vi "cam_tests.vi"() -> ()   [LabVIEW 2013]
uses:
  <vilib>/vision/driver/NI_Vision_Acquisition_Software.lvlib
  <vilib>/vision/Image Controls.llb/IMAQ Image.ctl
panel:
  out "All Images Out":T1[](array[plugin-control])
  in  "Number of Images":i32=10
  out "Image Out":T1(plugin-control)
  in  "Stop (F)":bool
  out "Image Out 2":T1(plugin-control)
  out "error out":errorcluster
  out "Image 3":T1(plugin-control)
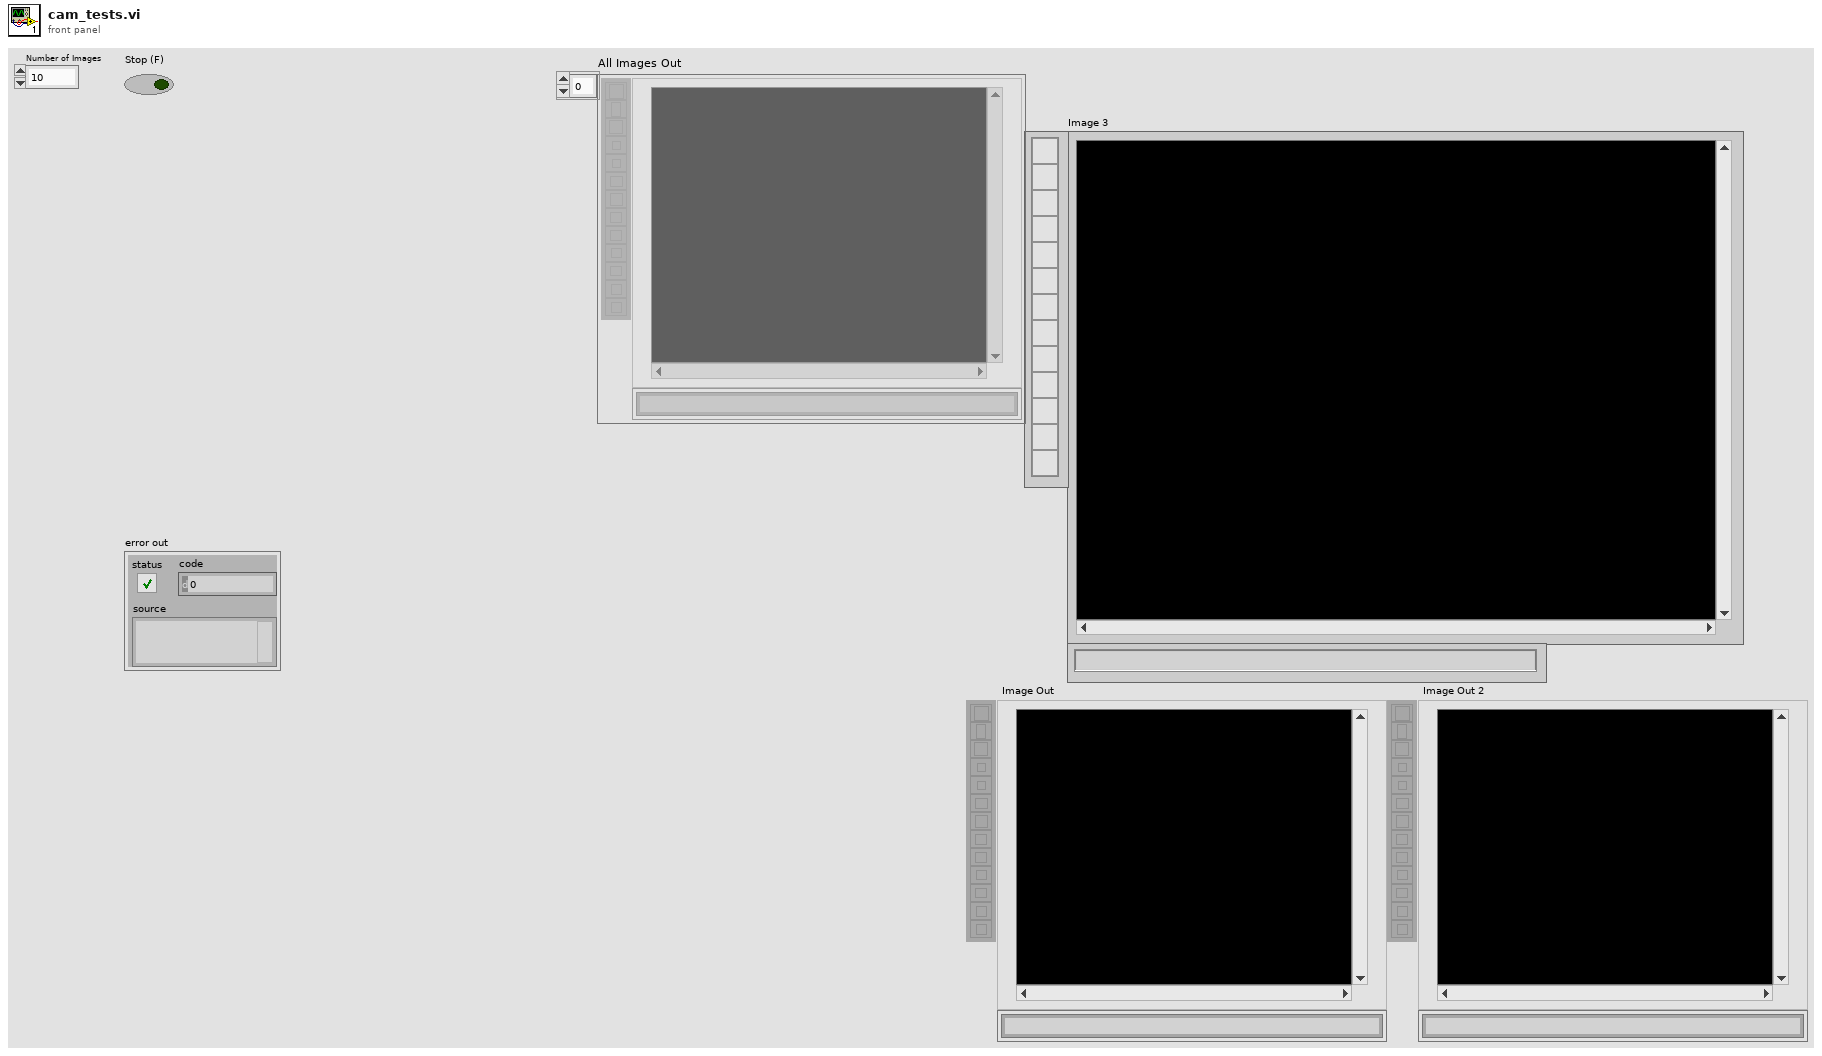
[diagram p1: front panel]
types:
  T1 = typedef "IMAQ Image.ctl" = refnum<image>
  T2 = typedef "IMAQdx.ctl" = refnum<k21>
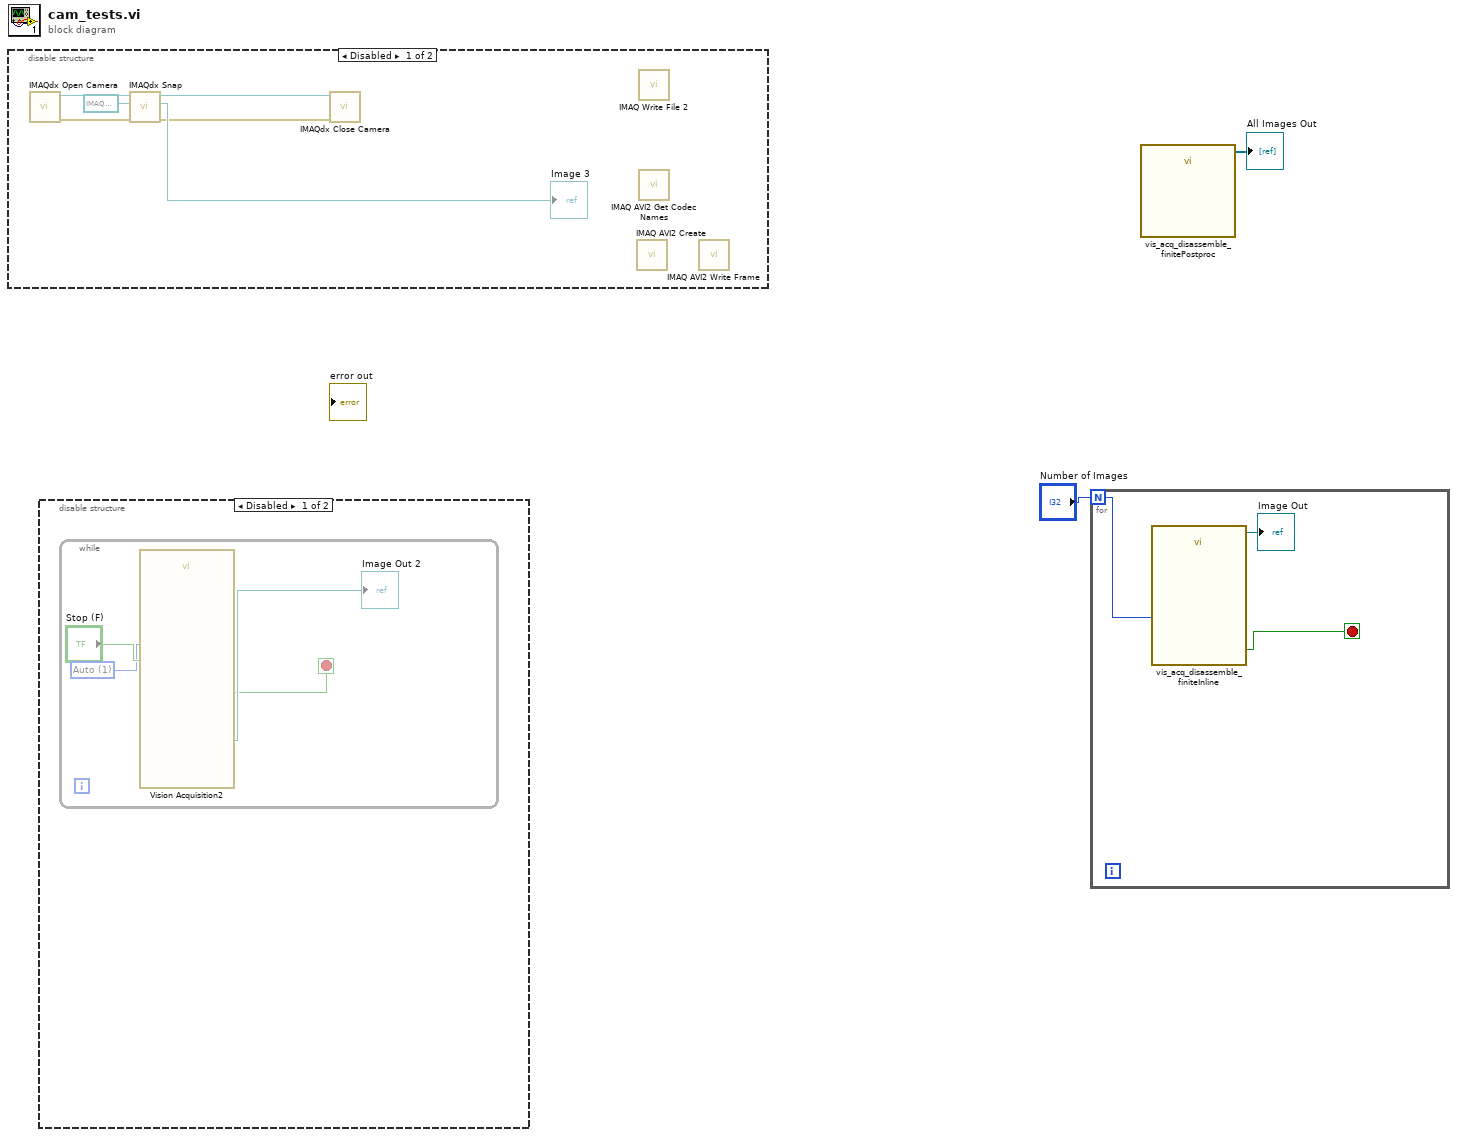
[diagram p0: block diagram]
diagram:
  n1 = disable-structure shown="Disabled" {
    frame Disabled {
      n2 = call <vilib>:"IMAQdx Open Camera.vi"() -> ("error out"=w6:errorcluster, "Session Out"=w7:T2)  [unwired: 10 in]
      n3 = call <vilib>:"IMAQdx Snap.vi"("error in"=w6, "Image In"=T1 refnum, "Session In"=w7) -> ("error out"=w4:errorcluster, "Image Out"=→"Image 3":T1, "Session Out"=w5:T2)  [unwired: 6 in]
      n4 = call <vilib>:"IMAQdx Close Camera.vi"("error in"=w4, "Session In"=w5) -> ()  [unwired: 9 in, 1 out]
      n5 = call "IMAQ AVI2 Create"() -> ()  [unwired: 10 in, 2 out]
      n6 = call-poly "IMAQ Write File 2"() -> ()  [unwired: 10 in, 2 out]
      n7 = call "IMAQ AVI2 Get Codec Names"() -> ()  [unwired: 10 in, 2 out]
      n8 = call "IMAQ AVI2 Write Frame"() -> ()  [unwired: 9 in, 3 out]
    }
    frame Enabled {
    }
  }
  n9 = disable-structure shown="Disabled" {
    frame Disabled {
      n10 = while {
        stop <- w10 stop-if-true
        w9 = u32 1 items=["Auto"=1, "Manual"=2] ("Focus::Mode")
        n11 = call "Vision Acquisition2"("Focus::Mode"=w9, "Stop (F)"="Stop (F)") -> ("Image Out"=→"Image Out 2":T1, "Stopped"=w10:bool)  [unwired: 20 in, 4 out]
      }
    }
    frame Enabled {
    }
  }
  n12 = for {
    N: "Number of Images" -> [w14]
    stop <- w13 stop-if-true
    n13 = call "vis_acq_disassemble_finiteInline.vi"("Number of Images"=w14) -> ("Image Out"=→"Image Out":T1, "Stopped"=w13:bool)  [unwired: 23 in, 2 out]
  }
  n14 = call "vis_acq_disassemble_finitePostproc.vi"() -> ("All Images Out"=→"All Images Out":T1[])  [unwired: 26 in, 1 out]
